vi "Init.vi"(6 "Simulated device name":string, 7 "simulated?":bool, 8 "error in (no error)":errorcluster, 9 "remote port":u16, 10 "address":string, 11 "TcpReader in":refnum<class "TcpReader.lvclass">) -> (0 "error out":errorcluster, 3 "TcpReader out":refnum<class "TcpReader.lvclass">)   [LabVIEW 2013, in "TcpReader.lvclass"]
doc: "Initializes the TCP reader as a client. The client will try to connect to the given adress and port and will reconnect if the connection fails"
uses:
  TcpReader.lvclass
  TcpReader.lvclass/TcpReader.ctl
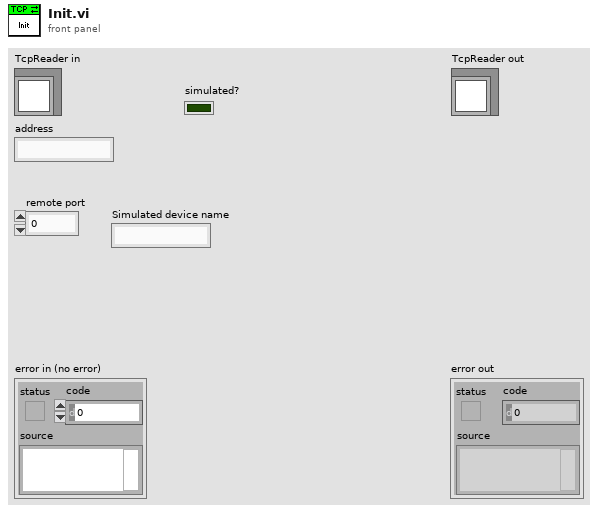
[diagram p1: front panel]
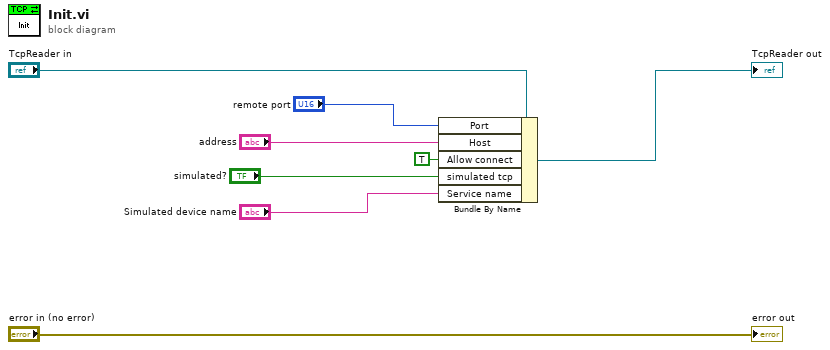
[diagram p0: block diagram]
diagram:
  n1 = Bundle By Name(cluster="TcpReader in", "Port"="remote port", "Host"="address", "Allow connect"=TRUE, "simulated tcp"="simulated?", "Service name"="Simulated device name") -> (→"TcpReader out":refnum<class "TcpReader.lvclass">)
  "error out" <- "error in (no error)"
